vi "Set TDMS File Property.vi"(5 "Property Value":variant, 7 "Property Name":string, 8 "error in (no error)":errorcluster, 11 "TDMS Log File in":refnum<class "TDMS Log File.lvclass">) -> (0 "error out":errorcluster, 3 "TDMS Log File out":refnum<class "TDMS Log File.lvclass">)   [LabVIEW 2012, in "Waveform Data Logger Engine.lvlib" / "TDMS Log File.lvclass"]
uses:
  TDMS Log File.lvclass
  TDMS Log File.lvclass/TDMS Log File.ctl
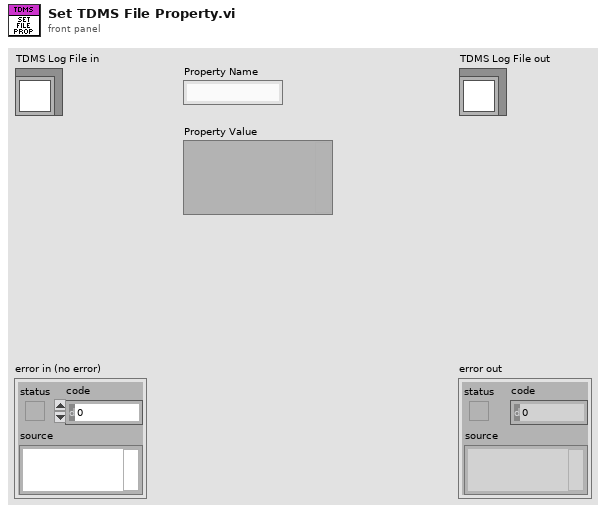
[diagram p1: front panel]
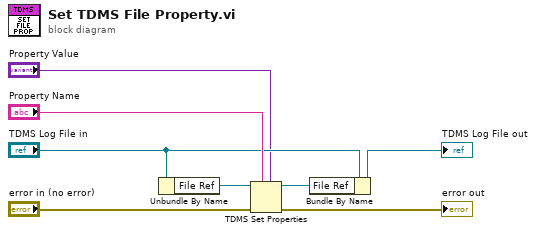
[diagram p0: block diagram]
diagram:
  n1 = Unbundle By Name("TDMS Log File in") -> ("File Ref"=w2:refnum<k34>)
  n2 = TDMS Set Properties(5:"Property Value", 7:"Property Name", 8:"error in (no error)", 11:w2) -> (0:→"error out":errorcluster, 3:w1:refnum<k34>)  [unwired: 2 in, 2 out]
  n3 = Bundle By Name(cluster="TDMS Log File in", "File Ref"=w1) -> (→"TDMS Log File out":refnum<class "TDMS Log File.lvclass">)
